vi "Rocket Dynamics (SubVI).vi"(4 "Rotation":T2, 5 "Position":T3, 6 "Time":T5, 7 "TVA":T1, 9 "Vehicle Param":T4, 10 "V_Wind [m/s]":dbl[][](array[numeric]), 11 "Data":dbl[][](array[numeric])) -> (0 "Aerodyn output":T6, 1 "ang_acc":dbl[](array[numeric]), 2 "M_alpha [rad/s^2], M_beta [rad/s^2]":T7, 3 "acc [m/s^2]":dbl[](array[numeric]))   [LabVIEW 2017]
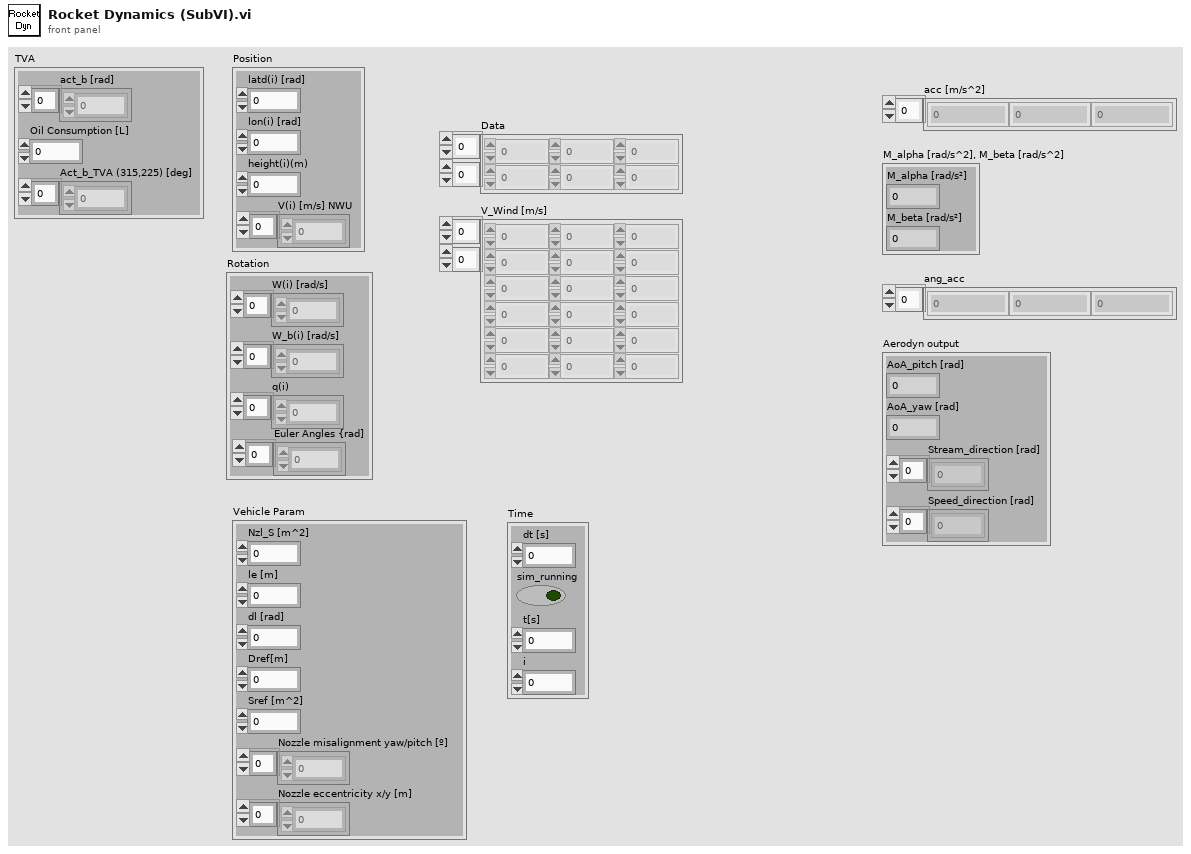
[diagram p1: front panel]
types:
  T1 = cluster{"act_b [rad]":dbl[], "Oil Consumption [L]":dbl, "Act_b_TVA (315,225) [deg]":dbl[]}
  T2 = cluster{"W(i) [rad/s]":dbl[], "W_b(i) [rad/s]":dbl[], "q(i)":dbl[], "Euler Angles {rad]":dbl[]}
  T3 = cluster{"latd(i) [rad]":dbl, "lon(i) [rad]":dbl, "height(i)(m)":dbl, "V(i) [m/s] NWU":dbl[]}
  T4 = cluster{"Nzl_S [m^2]":dbl, "le [m]":dbl, "dl [rad]":dbl, "Dref[m]":dbl, "Sref [m^2]":dbl, "Nozzle misalignment yaw/pitch [º]":dbl[], "Nozzle eccentricity x/y [m]":dbl[]}
  T5 = cluster{"dt [s]":dbl, "sim_running":bool, "t[s]":dbl, "i":i32}
  T6 = cluster{"AoA_pitch [rad]":dbl, "AoA_yaw [rad]":dbl, "Stream_direction [rad]":dbl[], "Speed_direction [rad]":dbl[]}
  T7 = cluster{"M_alpha [rad/s²]":dbl, "M_beta [rad/s²]":dbl}
  T8 = cluster{"Pdin [Pa]":dbl, "Patm [Pa]":dbl, "Temp [K]":dbl, "air flow velocity [m/s]":dbl}
  T9 = cluster{"AoA_pitch [rad]":dbl, "AoA_yaw [rad]":dbl, "Stream_direction [rad]":dbl[]}
  T10 = cluster{"FE_b [N]":dbl[], "FG [N]":dbl[], "FA [N]":dbl[], "Fco [N]":dbl[]}
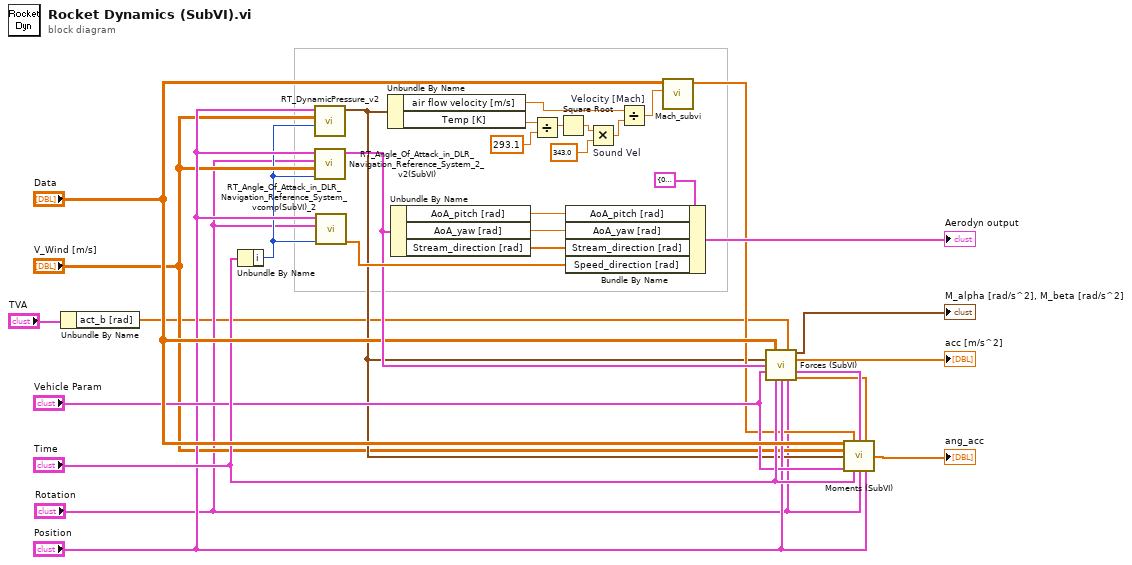
[diagram p0: block diagram]
diagram:
  n1 = Unbundle By Name("TVA") -> ("act_b [rad]"=w1:dbl[])
  n2 = Unbundle By Name("Time") -> ("i"=w9:i32)
  n3 = call "RT_DynamicPressure_v2.vi"("i"=w9, "V_wind [m/s]"="V_Wind [m/s]", "output cluster 2"="Position") -> ("output cluster"=w15:T8)  [unwired: 8 in]
  n4 = call "RT_Angle_Of_Attack_in_DLR_Navigation_Reference_System_2_v2(SubVI).vi"("i"=w9, "V_wind [m/s]"="V_Wind [m/s]", "Rotation"="Rotation", "output cluster 2"="Position") -> ("output cluster"=w24:T9)  [unwired: 7 in]
  n5 = call "RT_Angle_Of_Attack_in_DLR_Navigation_Reference_System_vcomp(SubVI)_2.vi"("i"=w9, "Rotation"="Rotation", "input cluster"="Position") -> ("Speed_direction [rad]"=w29:dbl[])  [unwired: 6 in, 2 out]
  n6 = Unbundle By Name(w15) -> ("air flow velocity [m/s]"=w11:dbl, "Temp [K]"=w18:dbl)
  n7 = Unbundle By Name(w24) -> ("AoA_pitch [rad]"=w25:dbl, "AoA_yaw [rad]"=w26:dbl, "Stream_direction [rad]"=w27:dbl[])
  n8 = Divide(x=w18, y=293.1) -> (x/y=w5:dbl)
  n9 = Square Root(x=w5) -> (sqrt(x)=w6:dbl)
  n10 = Bundle By Name(cluster=T6 {"AoA_pitch [rad]"=0.0, "AoA_yaw [rad]"=0.0, "Stream_direction [rad]"=[], "Speed_direction [rad]"=[]} ("output cluster"), "AoA_pitch [rad]"=w25, "AoA_yaw [rad]"=w26, "Stream_direction [rad]"=w27, "Speed_direction [rad]"=w29) -> (→"Aerodyn output":T6)
  n11 = Multiply "Sound Vel"(x=w6, y=343.0 ("x")) -> (x*y=w8:dbl)
  n12 = Divide "Velocity [Mach]"(x=w11, y=w8) -> (x/y=w10:dbl)
  n13 = call "Mach_subvi.vi"("Mach_IN"=w10, "Mach_File"="Data") -> ("OUT_Interp"=w16:dbl[])  [unwired: 9 in]
  n14 = call "Forces (SubVI).vi"("Data"="Data", "act_b"=w1, "Pdin [Pa], Patm [Pa], Temp [K], airflow velocity [m/s]"=w15, "AoA_pitch [rad], AoA_yaw [rad], Stream direction [rad]"=w24, "Vehicle Parameters"="Vehicle Param", "i, sim_running, t[s], dt[s]"="Time", "V(i) [m/s] NWU, latd(i) [rad], lon(i) [rad], height(i) [m]"="Position", "Rotation"="Rotation") -> ("M_alpha [rad/s^2], M_beta [rad/s^2]"=→"M_alpha [rad/s^2], M_beta [rad/s^2]":T7, "acc [m/s^2]"=→"acc [m/s^2]":dbl[], "FE_b [N], FG [N], FA [N], Fco[N]"=w13:T10, "FE [N]"=w12:dbl[])  [unwired: 4 in]
  n15 = call "Moments (SubVI).vi"("Data"="Data", "OUT_Interp"=w16, "FE_b [N], FG [N], FA [N], Fco[N]"=w13, "FE [N]"=w12, "V_Wind [m/s]"="V_Wind [m/s]", "Pdin [Pa], Patm [Pa], Temp [K], airflow velocity [m/s]"=w15, "Vehicle Parameters"="Vehicle Param", "i, sim_running, t[s], dt[s]"="Time", "Rotation"="Rotation", "V(i) [m/s] NWU, latd(i) [rad], lon(i) [rad], height(i) [m]"="Position") -> ("ang_acc"=→"ang_acc":dbl[])  [unwired: 5 in]
